vi "CheckHighTemp.vi"() -> ()   [LabVIEW 2012]
uses:
  <vilib>/addons/database/Auxilliary.llb/DB Tools Cursor Type.ctl
  <vilib>/addons/database/Connection.llb/DB Tools Open Connec (Path).vi
  <vilib>/addons/database/Connection.llb/Conn Execute.vi
  <vilib>/addons/database/Recordset.llb/Rec Fetch Recordset Data (R).vi
  <vilib>/addons/database/Recordset.llb/Rec Destroy - Connection.vi
  <vilib>/addons/database/_DB Variant To Data/Database Variant To Data.xnode
  <vilib>/addons/database/NI_Database_API.lvlib
  <vilib>/Utility/SMTP/NI_SMTPEmail.lvlib
panel:
  out "Output 2":string
  out "concatenated string 2":string
  out "concatenated string":string
  out "OK":bool
  out "before substring 3":string
  out "data":string
  out "recordset data":variant[][](array[variant])
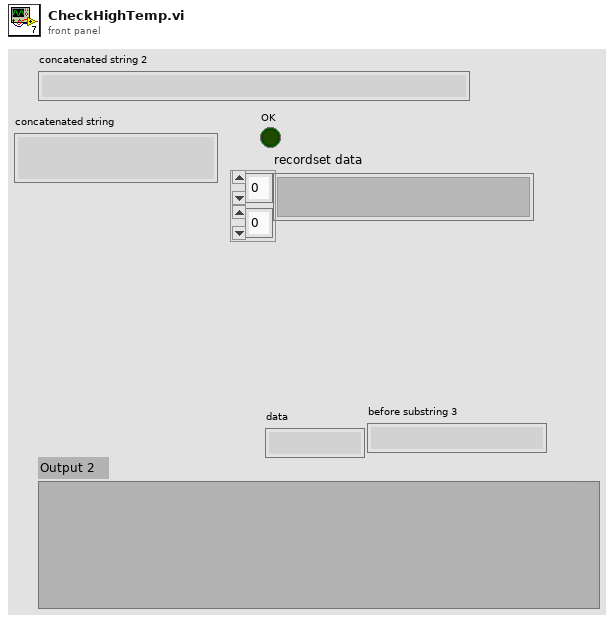
[diagram p1: front panel]
types:
  T1 = typedef "NI_Database_API.lvlib/DB Tools Cursor Type.ctl" = enum16{"forward-only", "keyset", "dynamic", "static"}
  T2 = typedef "NI_Database_API.lvlib/Conn ObjectReference.ctl" = refnum<k1>
  T3 = typedef "NI_Database_API.lvlib/Rec ObjectReference.ctl" = refnum<k1>
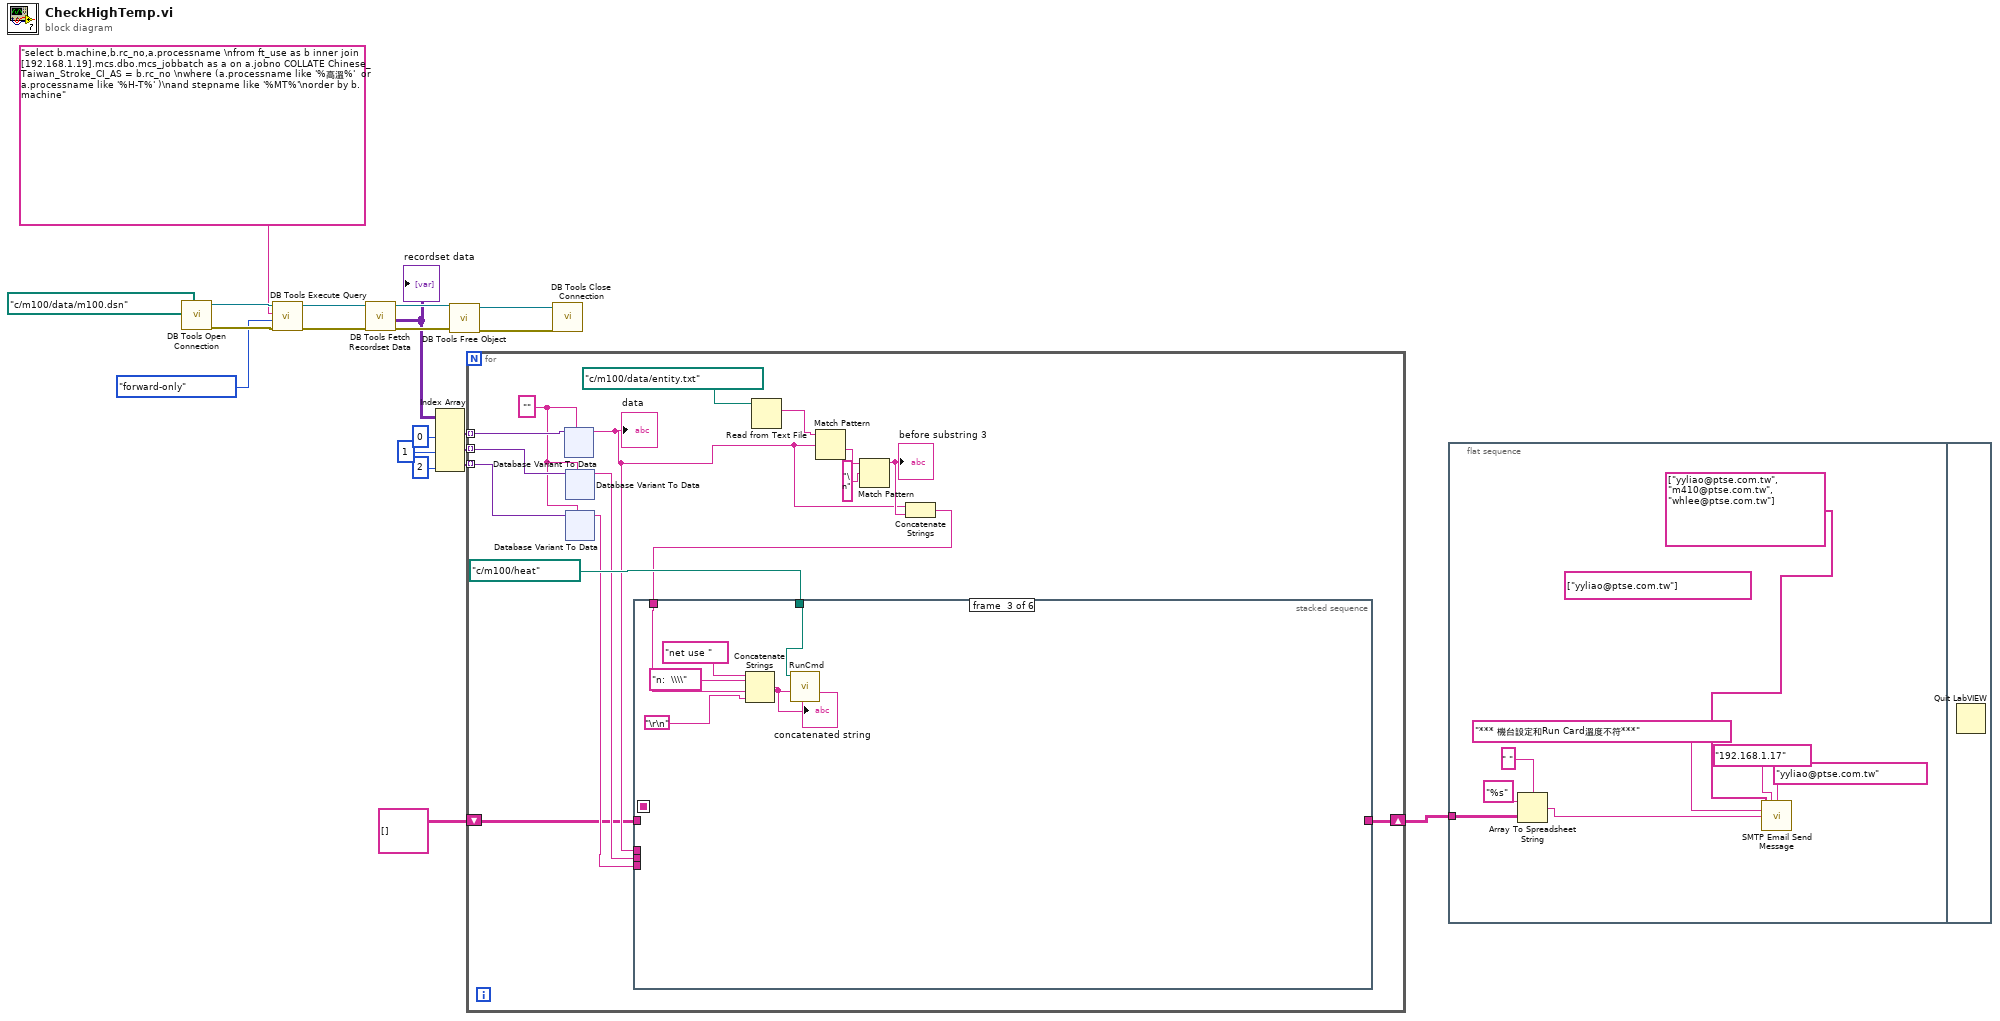
[diagram p0: block diagram]
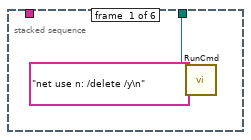
[diagram p2: hidden frame]
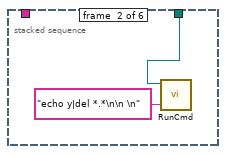
[diagram p3: hidden frame]
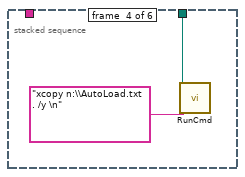
[diagram p4: hidden frame]
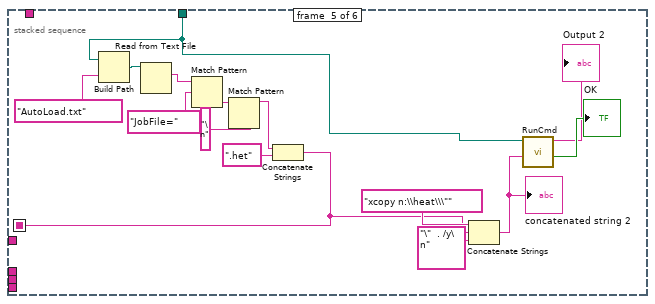
[diagram p5: hidden frame]
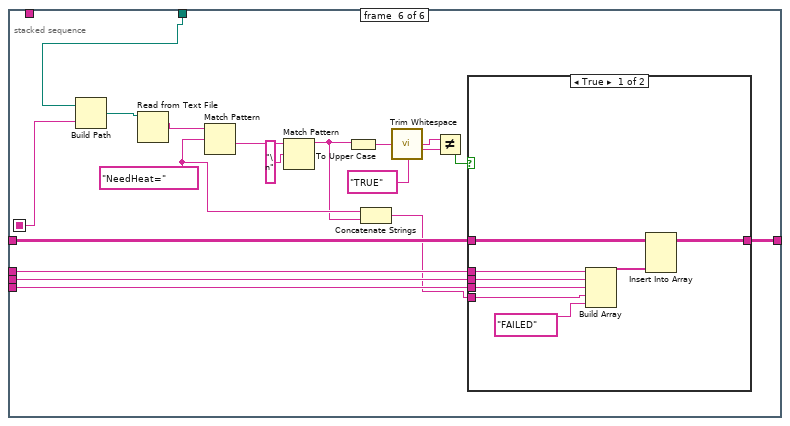
[diagram p6: hidden frame]
diagram:
  n1 = call-poly <vilib>:"DB Tools Open Connection.vi"("connection information"=path "c:/m100/data/m100.dsn") -> ("error out"=w16:errorcluster, "connection reference"=w20:T2)  [unwired: 7 in]
  n2 = call-poly <vilib>:"DB Tools Execute Query.vi"("error in (no error)"=w16, "cursor type"=DB_Tools_Cursor_Type."forward-only", "SQL query"="select b.machine,b.rc_no,a.processname \nfrom ft_use as b inner join [192.168.1.19].mcs.dbo.mcs_jobbatch as a on a.jobno COLLATE Chinese_Taiwan_Stroke_CI_AS = b.rc_no \nwhere (a.processname like '%高溫%'  or  a.processname like '%H-T%' )\nand stepname like '%MT%'\norder by b.machine", "connection reference"=w20) -> ("error out"=w15:errorcluster, "recordset reference"=w19:T3)  [unwired: 4 in]
  n3 = call-poly <vilib>:"DB Tools Fetch Recordset Data.vi"("error in (no error)"=w15, "recordset reference"=w19) -> ("error out"=w14:errorcluster, "recordset data"=w9:variant[][], "recordset reference out"=w18:T3)  [unwired: 3 in]
  "recordset data" <- w9
  n4 = Index Array(array=w9, index (col) #1=0 ("disabled index (col)"), index (col) #2=1 ("index (col)"), index (col) #3=2 ("index (col)")) -> (element #1=w7:variant[], element #2=w4:variant[], element #3=w3:variant[])  [unwired: 3 in]
  n5 = call-poly <vilib>:"DB Tools Free Object.vi"("error in (no error)"=w14, "recordset reference"=w18) -> ("error out"=w13:errorcluster, "connection reference"=w17:T2)  [unwired: 8 in]
  n6 = for {
    tunnel: w7 -> [w36] mode=indexing
    tunnel: w4 -> [w28] mode=indexing
    tunnel: w3 -> [w27] mode=indexing
    shift-right: [w22] -> w1
    shift-left: string[][] [] ("array") -> [w21]
    w26 = ""
    n7 = xnode "Database Variant To Data"("database variant"=w36, "type"=w26) -> ("data"=w25:string)  [unwired: 1 in, 1 out]
    "data" <- w25
    n8 = xnode "Database Variant To Data"("database variant"=w28, "type"=w26) -> ("data"=w24:string)  [unwired: 1 in, 1 out]
    n9 = xnode "Database Variant To Data"("database variant"=w27, "type"=w26) -> ("data"=w23:string)  [unwired: 1 in, 1 out]
    n10 = Read from Text File(file (use dialog)=path "c:/m100/data/entity.txt") -> (text=w34:string)  [unwired: 3 in, 3 out]
    n11 = Match Pattern(string=w34, regular expression=w25) -> (after substring=w33:string)  [unwired: 1 in, 3 out]
    n12 = Match Pattern(string=w33, regular expression="\n") -> (before substring=w30:string)  [unwired: 1 in, 3 out]
    "before substring 3" <- w30
    n13 = Concatenate Strings(w25, w30) -> (w29:string)
    n14 = stacked-sequence {
      seq-local: [_ _ _ _ w113 _] -> [_ _ _ _ _ w140]
      tunnel: path "c:/m100/heat" ("working directory") -> [w101 w104 w105 w111 w119 w142]
      tunnel: w29 -> [_ _ w106 _ _ _]
      tunnel: w25 -> [_ _ _ _ _ w135]
      tunnel: w24 -> [_ _ _ _ _ w134]
      tunnel: w23 -> [_ _ _ _ _ w133]
      tunnel: [_ _ _ _ _ w132] -> w22
      tunnel: w21 -> [_ _ _ _ _ w131]
      frame #0 {
        n15 = call "RunCmd.vi"("Cmd String"="net use n: /delete /y\n" ("string"), "working directory"=w101) -> ()  [unwired: 8 in, 2 out]
      }
      frame #1 {
        n16 = call "RunCmd.vi"("Cmd String"="echo y|del *.*\n\n \n" ("standard input"), "working directory"=w104) -> ()  [unwired: 8 in, 2 out]
      }
      frame #2 {
        n17 = Concatenate Strings("net use " ("string"), "n:  \\\\" ("string"), w106, "\r\n") -> (w110:string)
        "concatenated string" <- w110
        n18 = call "RunCmd.vi"("Cmd String"=w110, "working directory"=w105) -> ()  [unwired: 8 in, 2 out]
      }
      frame #3 {
        n19 = call "RunCmd.vi"("Cmd String"="xcopy n:\\AutoLoad.txt . /y \n" ("standard input"), "working directory"=w111) -> ()  [unwired: 8 in, 2 out]
      }
      frame #4 {
        n20 = Build Path(base path=w119, name or relative path="AutoLoad.txt") -> (appended path=w120:path)
        n21 = Read from Text File(file (use dialog)=w120) -> (text=w127:string)  [unwired: 3 in, 3 out]
        n22 = Match Pattern(string=w127, regular expression="JobFile=") -> (after substring=w125:string)  [unwired: 1 in, 3 out]
        n23 = Match Pattern(string=w125, regular expression="\n") -> (before substring=w123:string)  [unwired: 1 in, 3 out]
        n24 = Concatenate Strings(w123, ".het" ("string")) -> (w113:string)
        n25 = Concatenate Strings("xcopy n:\\heat\\\"" ("standard input"), w113, "\"  . /y\n" ("string")) -> (w116:string)
        "concatenated string 2" <- w116
        n26 = call "RunCmd.vi"("Cmd String"=w116, "working directory"=w119) -> ("OK"=→"OK":bool, "Output"=→"Output 2":string)  [unwired: 8 in]
      }
      frame #5 {
        w130 = "NeedHeat=" ("regular expression")
        n27 = Build Path(base path=w142, name or relative path=w140) -> (appended path=w141:path)
        n28 = Read from Text File(file (use dialog)=w141) -> (text=w145:string)  [unwired: 3 in, 3 out]
        n29 = Match Pattern(string=w145, regular expression=w130) -> (after substring=w144:string)  [unwired: 1 in, 3 out]
        n30 = Match Pattern(string=w144, regular expression="\n") -> (before substring=w129:string)  [unwired: 1 in, 3 out]
        n31 = To Upper Case(1:w129) -> (0:w139:string)
        n32 = Concatenate Strings(w130, w129) -> (w128:string)
        n33 = call <vilib>:"Trim Whitespace.vi"("string"=w139) -> ("trimmed string"=w138:string)  [unwired: 1 in]
        n34 = Not Equal?(x=w138, y="TRUE") -> (x != y?=w136:bool)
        n35 = case shown="True" w136 {
          tunnel: w135 -> [w153 _]
          tunnel: w134 -> [w152 _]
          tunnel: w133 -> [w151 _]
          tunnel: [w150 w154] -> w132
          tunnel: w131 -> [w149 w154]
          tunnel: w128 -> [w147 _]
          frame True {
            n36 = Build Array(w153, w152, w151, w147, "FAILED" ("string")) -> (w148:string[])
            n37 = Insert Into Array(array=w149, new element=w148) -> (w150:string[][])  [unwired: 2 in]
          }
          frame False {
          }
        }
      }
    }
  }
  n38 = call <vilib>:"DB Tools Close Connection.vi"("error in (no error)"=w13, "connection reference"=w17) -> ()  [unwired: 5 in, 1 out]
  n39 = flat-sequence {
    tunnel: w1 -> [w192]
    frame #0 {
      (unwired) string[] ["yyliao@ptse.com.tw"] ("recipients")
      n40 = Array To Spreadsheet String(delimiter (Tab)=" ", array=w192, 3:"%s" ("format string")) -> (spreadsheet string=w188:string)
      n41 = call <vilib>:"SMTP Email Send Message.vi"("recipients"=string[] ["yyliao@ptse.com.tw", "m410@ptse.com.tw", "whlee@ptse.com.tw"], "mail server"="192.168.1.17", "return address"="yyliao@ptse.com.tw", "subject ([No Subject])"="*** 機台設定和Run Card溫度不符***", "message"=w188) -> ()  [unwired: 9 in, 2 out]
    }
    frame #1 {
      n42 = Quit LabVIEW() -> ()  [unwired: 1 in]
    }
  }
